vi "Test Serializer.Text.issue10.vi"(8 "error in (no error)":errorcluster) -> (0 "error out":errorcluster)   [LabVIEW 2013]
uses:
  source/Serializer.PlainText/Serializer.PlainText.lvclass
  <vilib>/addons/_JKI Toolkits/Caraya/classes/Assert/Assert Not Error.vi
  <vilib>/addons/_JKI Toolkits/Caraya/classes/Assert/Assert.lvclass
  source/Serializer/Serializer.lvclass
  <vilib>/addons/_JKI Toolkits/Caraya/classes/Test/Test.lvclass
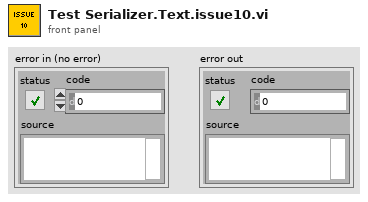
[diagram p1: front panel]
types:
  T1 = cluster{"String":string, "Array":cluster{"Array":dbl[], "String":string}[]}[]
  T2 = cluster{"Array":cluster{"Array":dbl[], "String":string}[]}
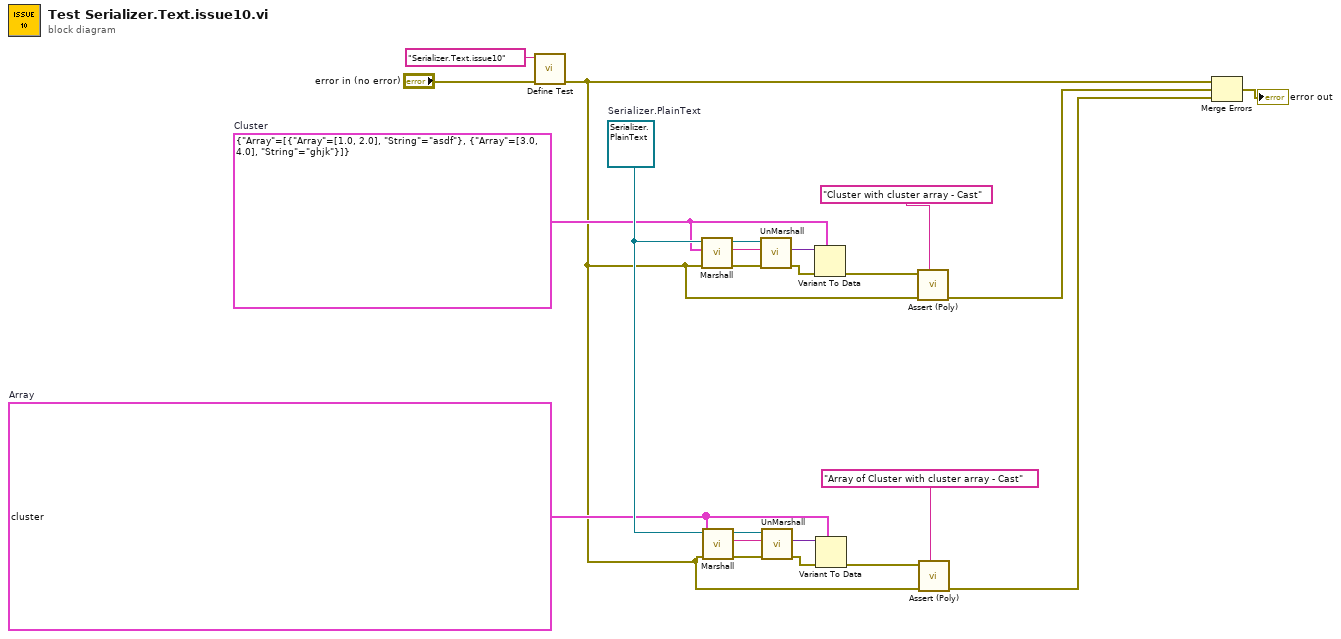
[diagram p0: block diagram]
diagram:
  w4 = T1 [{"String"="asdf", "Array"=[{"Array"=[1.0, 2.0], "String"="zxcv"}, {"Array"=[3.0, 4.0], "String"="bnm"}]}, {"String"="ghjk", "Array"=[{"Array"=[5.0, 6.0], "String"="qwer"}, {"Array"=[7.0, 8.0], "String"="tyui"}]}]  # Array
  w6 = T2 {"Array"=[{"Array"=[1.0, 2.0], "String"="asdf"}, {"Array"=[3.0, 4.0], "String"="ghjk"}]}  # Cluster
  w7 = refnum<class "Serializer.PlainText.lvclass"> refnum  # Serializer.PlainText
  n1 = call <vilib>:"Define Test.vi"("error in (no error)"="error in (no error)", "Label (VI Title)"="Serializer.Text.issue10") -> ("error out"=w1:errorcluster)  [unwired: 9 in]
  n2 = call "Marshall.vi"("error in (no error)"=w1, "Variant"=w6, "Serializer in"=w7) -> ("error out"=w18:errorcluster, "String"=w20:string, "Serializer out"=w19:refnum<class "Serializer.PlainText.lvclass">)  [unwired: 6 in]
  n3 = call "Marshall.vi"("error in (no error)"=w1, "Variant"=w4, "Serializer in"=w7) -> ("error out"=w13:errorcluster, "String"=w11:string, "Serializer out"=w12:refnum<class "Serializer.PlainText.lvclass">)  [unwired: 6 in]
  n4 = call "UnMarshall.vi"("error in (no error)"=w18, "String"=w20, "Serializer in"=w19) -> ("error out"=w9:errorcluster, "Variant"=w17:variant)  [unwired: 6 in, 1 out]
  n5 = call "UnMarshall.vi"("error in (no error)"=w13, "String"=w11, "Serializer in"=w12) -> ("error out"=w8:errorcluster, "Variant"=w14:variant)  [unwired: 6 in, 1 out]
  n6 = Variant To Data(error in=w9, type=w6, Variant=w17) -> (error out=w16:errorcluster)  [unwired: 1 out]
  n7 = Variant To Data(error in=w8, type=w4, Variant=w14) -> (error out=w15:errorcluster)  [unwired: 1 out]
  n8 = call-poly <vilib>:"Assert (Poly).vi"("Label"="Cluster with cluster array - Cast", "error in (no error)"=w1, "Not Error?"=w16) -> ("error out"=w5:errorcluster)  [unwired: 8 in]
  n9 = call-poly <vilib>:"Assert (Poly).vi"("Label"="Array of Cluster with cluster array - Cast", "error in (no error)"=w1, "Not Error?"=w15) -> ("error out"=w3:errorcluster)  [unwired: 8 in]
  n10 = Merge Errors(w1, w5, w3) -> (→"error out":errorcluster)
